vi "SS_Create_File.vi"(6 "Main Cluster IN":T1, 8 "Error In":errorcluster, 11 "Info In":string="\nWaiting for TimerScope Trigger\n- IN: SS TimerScope Trigger\n- OUT: SET SS ThermoRec Received Trigger\nPulse Number is 231123\nPulse Type is 4\n\nDuration (s) is  2.000000\nDelay (s)  is  1.000000\nScan Period (ms) is  15\nNumber of Samples is  134\n\nDelay Started\nDelay Complete\nExternal Measurement of Delay (s): 1.000000\nACQUIRING DATA") -> (0 "Error Out":errorcluster, 3 "Info Out":string="\nWaiting for TimerScope Trigger\n- IN: SS TimerScope Trigger\n- OUT: SET SS ThermoRec Received Trigger\nPulse Number is 231123\nPulse Type is 4\n\nDuration (s) is  2.000000\nDelay (s)  is  1.000000\nScan Period (ms) is  15\nNumber of Samples is  134\n\nDelay Started\nDelay Complete\nExternal Measurement of Delay (s): 1.000000\nACQUIRING DATA", 4 "Main Cluster OUT":T1)   [LabVIEW 2016]
uses:
  Control/Control_Main.ctl
  Control/Control_ModuleArray.ctl
panel:
  in  "Tab Control":enum32{"IN", "OUT", "SubVI Info"}(tab)
  out "Array - String":string[][](array[string])
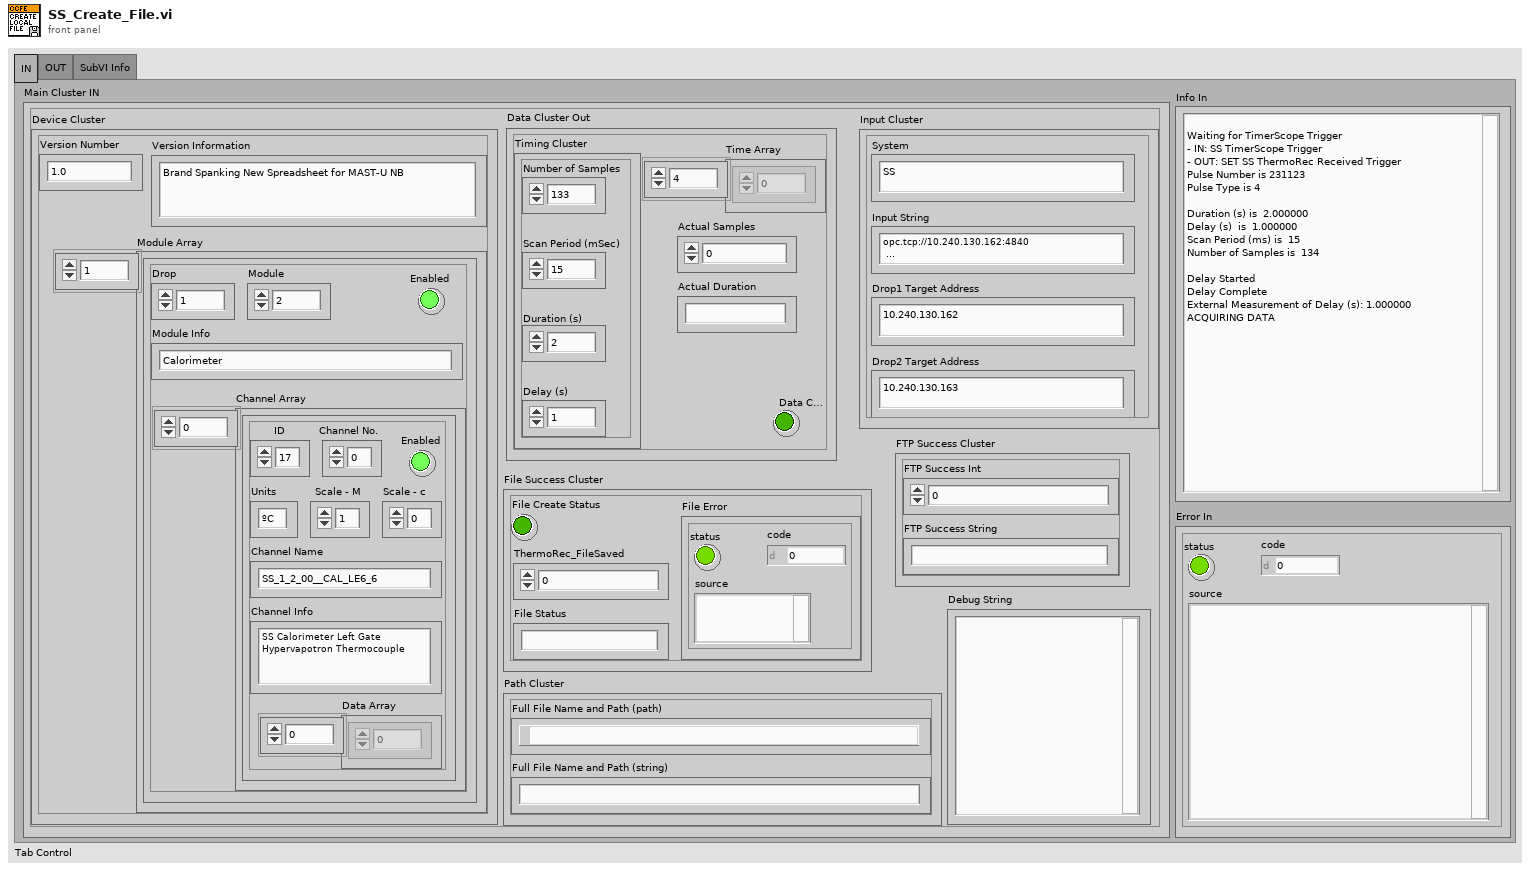
[diagram p1: front panel]
types:
  T1 = typedef "Control_Main.ctl" = cluster{"Device Cluster":cluster{"Module Array":T2, "Version Number":string, "Version Information":string}, "Input Cluster":cluster{"Input String":string, "Drop1 Target Address":string, "Drop2 Target Address":string, "System":string}, "Data Cluster Out":cluster{"Timing Cluster":cluster{"Number of Samples":i32, "Scan Period (mSec)":u32, "Duration (s)":dbl, "Delay (s)":dbl}, "Time Array":dbl[], "Actual Samples":i32, "Actual Duration":string, "Data Collection Error":bool}, "Path Cluster":cluster{"Full File Name and Path (path)":path, "Full File Name and Path (string)":string}, "File Success Cluster":cluster{"ThermoRec_FileSaved":i32, "File Create Status":bool, "File Error":errorcluster, "File Status":string}, "FTP Success Cluster":cluster{"FTP Success Int":i32, "FTP Success String":string}, "Debug String":string}
  T2 = typedef "Control_ModuleArray.ctl" = cluster{"Drop":i32, "Module":i32, "Module Info":string, "Enabled":bool, "Channel Array":cluster{"ID":i32, "Channel No.":i32, "Enabled":bool, "Channel Name":string, "Channel Info":string, "Units":string, "Scale - M":dbl, "Scale - c":dbl, "Data Array":dbl[]}[]}[]
  T3 = cluster{"ID":i32, "Channel No.":i32, "Enabled":bool, "Channel Name":string, "Channel Info":string, "Units":string, "Scale - M":dbl, "Scale - c":dbl, "Data Array":dbl[]}[]
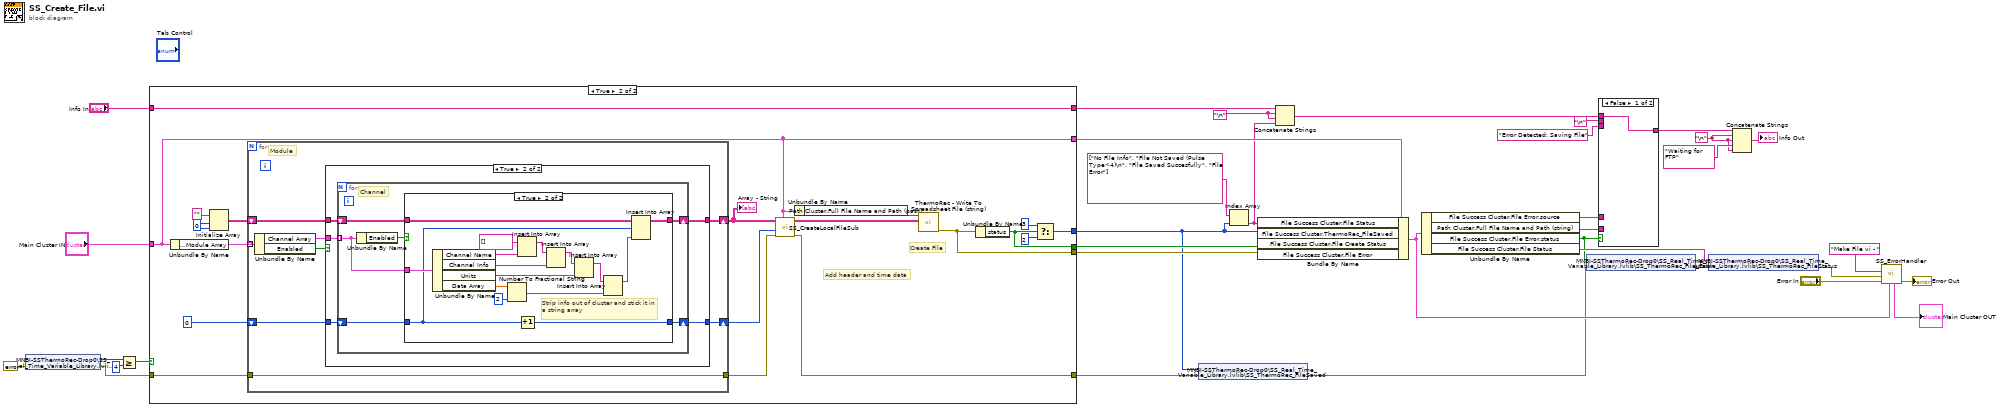
[diagram p0: block diagram]
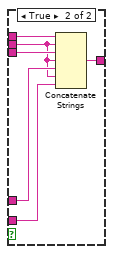
[diagram p2: hidden frame]
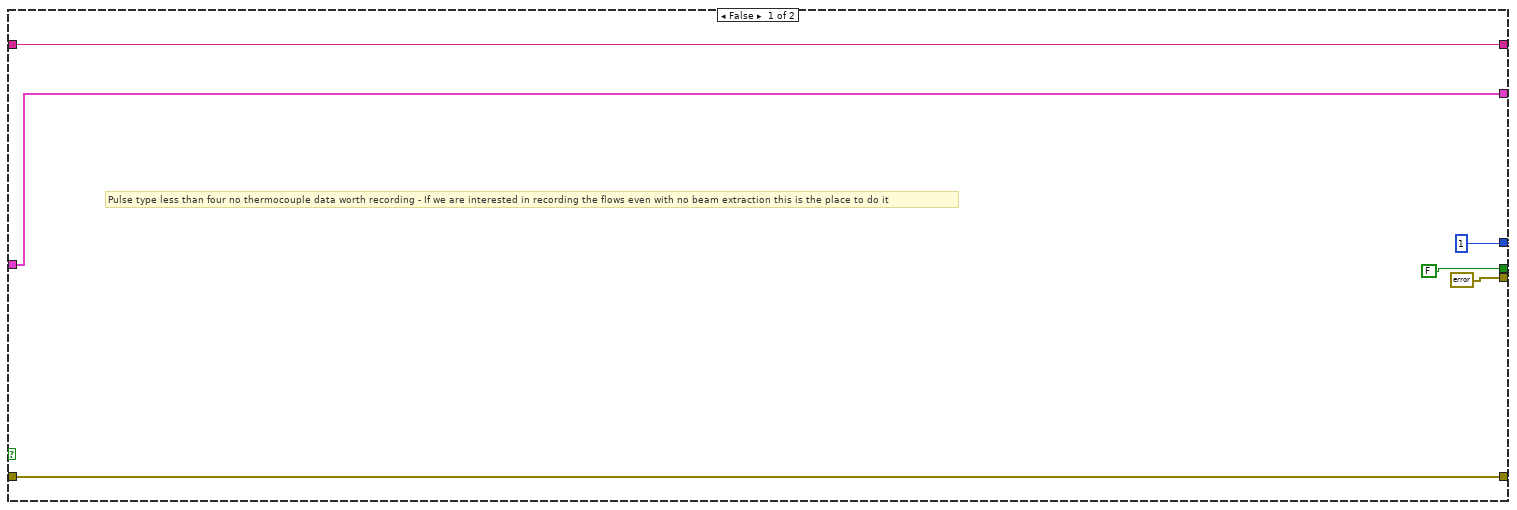
[diagram p3: hidden frame]
diagram:
  w6 = "\n"
  w7 = "\n"
  n1 = shared-variable "MNBI-SSThermoRec-Drop0\\SS_Real_Time_Variable_Library.lvlib\\SS_Pulse_Type"(error in=errorcluster {"status"=FALSE, "code"=0, "source"=""} ("error constant")) -> (w24:i32, error out=w23:errorcluster)
  n2 = Greater Or Equal?(x=w24, y=4) -> (x >= y?=w34:bool)
  n3 = case shown="True" w34 {
    tunnel: "Main Cluster IN" -> [w38 w48]
    tunnel: [errorcluster {"status"=FALSE, "code"=0, "source"=""} ("File Error") w45] -> w19
    tunnel: [1 w54] -> w2
    tunnel: "Info In" -> [w39 w53]
    tunnel: [w39 w53] -> w33
    tunnel: [w38 w48] -> w21
    tunnel: w23 -> [w36 w52]
    tunnel: [FALSE ("File Create Status") w50] -> w18
    tunnel: [w36 w43] -> w4
    frame False {
      # "Pulse type less than four no thermocouple data worth recording - If we are interested in recording the flows even with no beam extraction this is the place to do it"
    }
    frame True {
      w58 = 0
      # "Add header and time data"
      # "Create File"
      n4 = Unbundle By Name(w48) -> ("Device Cluster.Module Array"=w42:T2)
      n5 = Initialize Array("", w58, w58) -> (w57:string[][])
      n6 = for {
        tunnel: w42 -> [w66] mode=indexing
        shift-right: [w64] -> w47
        shift-left: 0 -> [w65]
        shift-right: [w62] -> w44
        shift-left: w57 -> [w63]
        tunnel: [w61] -> w46
        tunnel: w52 -> [w61]
        # "Module"
        n7 = Unbundle By Name(w66) -> ("Channel Array"=w68:T3, "Enabled"=w67:bool)
        n8 = case shown="True" w67 {
          tunnel: w68 -> [_ w75]
          tunnel: w65 -> [w70 w74]
          tunnel: [w70 w71] -> w64
          tunnel: w63 -> [w69 w73]
          tunnel: [w69 w72] -> w62
          frame False {
            # "The module is not enabled so ignore"
          }
          frame True {
            n9 = for {
              tunnel: w75 -> [w80] mode=indexing
              shift-right: [w76] -> w72
              shift-left: w73 -> [w78]
              shift-right: [w77] -> w71
              shift-left: w74 -> [w79]
              # "Channel"
              n10 = Unbundle By Name(w80) -> ("Enabled"=w81:bool)
              n11 = case shown="True" w81 {
                tunnel: w80 -> [_ w99]
                tunnel: w79 -> [w83 w84]
                tunnel: [w83 w85] -> w77
                tunnel: w78 -> [w82 w86]
                tunnel: [w82 w87] -> w76
                frame False {
                  # "The Channel is not enabled so ignore"
                }
                frame True {
                  # "Strip info out of cluster and stick it in a string array"
                  n12 = Unbundle By Name(w99) -> ("Channel Name"=w95:string, "Channel Info"=w93:string, "Units"=w91:string, "Data Array"=w98:dbl[])
                  n13 = Number To Fractional String(number=w98, precision (6)=i16 2) -> (F-format string=w89:string[])  [unwired: 2 in]
                  n14 = Insert Into Array(array=string[] [], new element=w95) -> (w94:string[])  [unwired: 1 in]
                  n15 = Increment(x=w84) -> (x+1=w85:i32)
                  n16 = Insert Into Array(array=w94, new element=w93) -> (w92:string[])  [unwired: 1 in]
                  n17 = Insert Into Array(array=w92, new element=w91) -> (w90:string[])  [unwired: 1 in]
                  n18 = Insert Into Array(array=w90, new element=w89) -> (w88:string[])  [unwired: 1 in]
                  n19 = Insert Into Array(array=w86, index (row)=w84, new element=w88) -> (w87:string[][])  [unwired: 1 in]
                }
              }
            }
          }
        }
      }
      "Array - String" <- w44
      n20 = call "SS_CreateLocalFileSub.vi"("Main Cluster IN"=w48, "Error IN"=w46, "Number of Channels"=w47, "Data Array IN"=w44) -> ("Error OUT"=w43:errorcluster, "Data Array OUT"=w49:string[][])  [unwired: 6 in]
      n21 = Unbundle By Name(w48) -> ("Path Cluster.Full File Name and Path (path)"=w51:path)
      n22 = call "ThermoRec - Write To Spreadsheet File (string).vi"("2D data"=w49, "file path (dialog if empty)"=w51) -> ("Write to Spreadsheet File Error"=w45:errorcluster)  [unwired: 6 in, 1 out]
      n23 = Unbundle By Name(w45) -> ("status"=w50:bool)
      n24 = Select(t=3, s=w50, f=2 ("t")) -> (s? t:f=w54:i32)
    }
  }
  n25 = shared-variable "MNBI-SSThermoRec-Drop0\\SS_Real_Time_Variable_Library.lvlib\\SS_ThermoRec_FileSaved"(w2, error in=w4) -> (error out=w3:errorcluster)
  n26 = Index Array(array=string[] ["No File Info", "File Not Saved (Pulse Type<4)\n", "File Saved Succesfully", "File Error"], index=w2) -> (element=w5:string)
  n27 = Bundle By Name(cluster=w21, "File Success Cluster.File Status"=w5, "File Success Cluster.ThermoRec_FileSaved"=w2, "File Success Cluster.File Create Status"=w18, "File Success Cluster.File Error"=w19) -> (w10:T1)
  n28 = Concatenate Strings(w33, w7, w7, w5) -> (w26:string)
  n29 = Unbundle By Name(w10) -> ("File Success Cluster.File Error.source"=w28:string, "Path Cluster.Full File Name and Path (string)"=w25:string, "File Success Cluster.File Error.status"=w1:bool, "File Success Cluster.File Status"=w20:string)
  n30 = shared-variable "MNBI-SSThermoRec-Drop0\\SS_Real_Time_Variable_Library.lvlib\\SS_ThermoRec_File_Error"(w1, error in=w3) -> (error out=w30:errorcluster)
  n31 = case shown="False" w1 {
    tunnel: w26 -> [w100 w106]
    tunnel: [w100 w101] -> w32
    tunnel: "\n" -> [_ w103]
    tunnel: w28 -> [_ w104]
    tunnel: "Error Detected: Saving File" -> [_ w105]
    tunnel: w25 -> [_ w102]
    frame False {
    }
    frame True {
      n32 = Concatenate Strings(w106, w103, w105, w103, w104, w103, w102) -> (w101:string)
    }
  }
  n33 = shared-variable "MNBI-SSThermoRec-Drop0\\SS_Real_Time_Variable_Library.lvlib\\SS_ThermoRec_FileStatus"(w20, error in=w30) -> (error out=w9:errorcluster)
  n34 = Concatenate Strings(w32, w6, w6, "Waiting for FTP", w6) -> (→"Info Out":string)
  n35 = call "SS_ErrorHandler.vi"("Main Cluster IN"=w10, "Error In"="Error In", "SubVI Error"=w9, "SubVI Name"="Make File vi - ") -> ("Error Out"=→"Error Out":errorcluster, "Main Cluster OUT"=→"Main Cluster OUT":T1)  [unwired: 5 in, 1 out]
